vi "GUI_BELLA_CAP_PLC.vi"() -> ()   [LabVIEW 2013]
panel:
  out "OutPos_Sen":bool
  out "InPos_Sen":bool
  out "OutPos_Ctrl":bool
  out "InPos_Ctrl":bool
  in  "MoveOut":bool
  in  "stop":bool
  out "OutPos":bool
  out "InPos":bool
  in  "MoveIn":bool
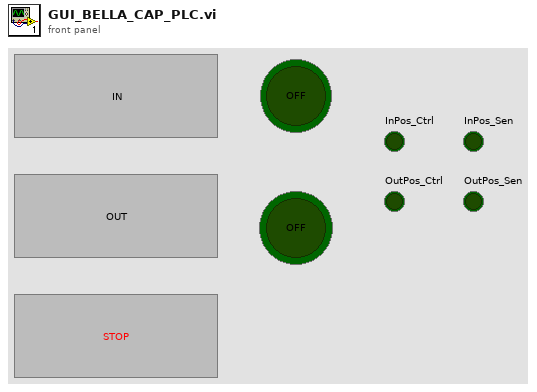
[diagram p1: front panel]
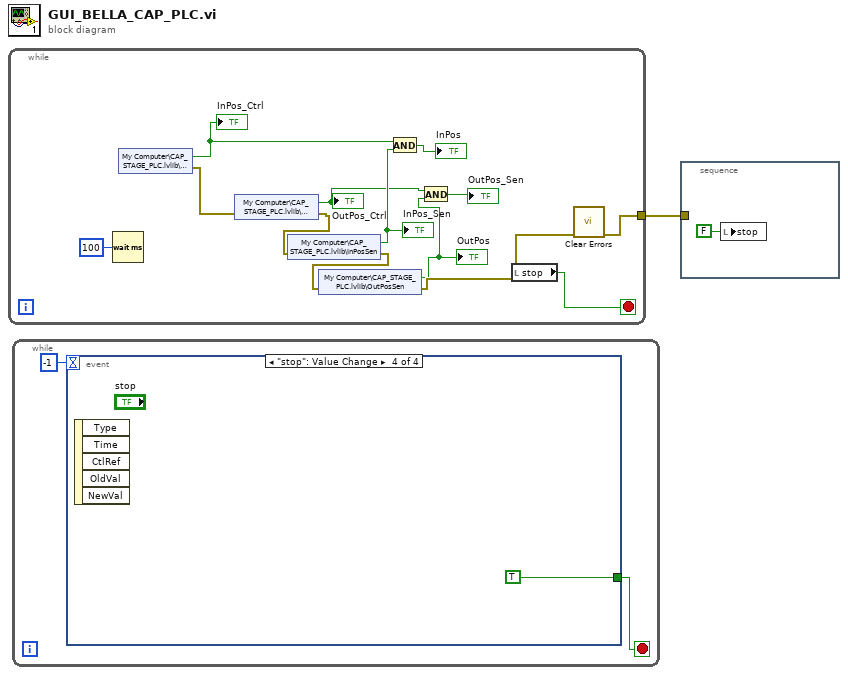
[diagram p0: block diagram]
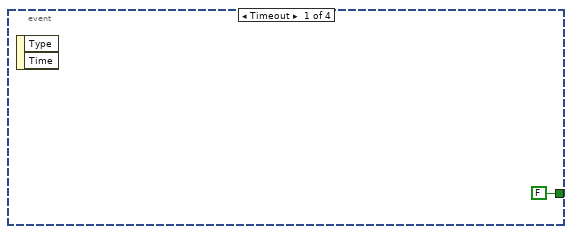
[diagram p2: hidden frame]
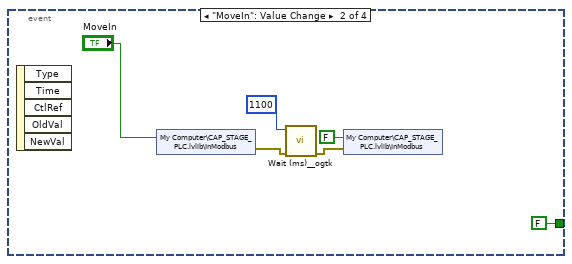
[diagram p3: hidden frame]
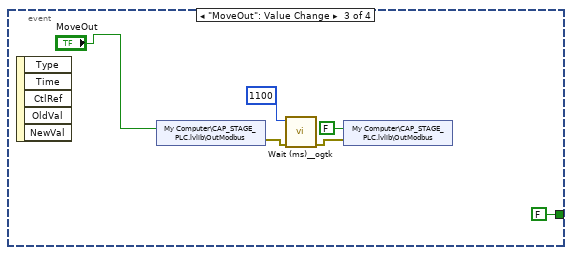
[diagram p4: hidden frame]
diagram:
  n1 = while {
    tunnel: [w11] -> w1
    stop <- w14 stop-if-true
    n2 = Wait (ms)(milliseconds to wait=u32 100) -> ()  [unwired: 1 out]
    n3 = shared-variable "My Computer\\CAP_STAGE_PLC.lvlib\\InPos"() -> (w6:bool, error out=w12:errorcluster)  [unwired: 1 in]
    "InPos_Ctrl" <- w6
    n4 = shared-variable "My Computer\\CAP_STAGE_PLC.lvlib\\OutPos"(error in=w12) -> (w3:bool, error out=w10:errorcluster)
    "OutPos_Ctrl" <- w3
    n5 = shared-variable "My Computer\\CAP_STAGE_PLC.lvlib\\InPosSen"(error in=w10) -> (w7:bool, error out=w9:errorcluster)
    "InPos_Sen" <- w7
    n6 = shared-variable "My Computer\\CAP_STAGE_PLC.lvlib\\OutPosSen"(error in=w9) -> (w4:bool, error out=w8:errorcluster)
    "OutPos" <- w4
    n7 = And(x=w6, y=w7) -> (x .and. y?=→"InPos":bool)
    n8 = And(x=w3, y=w4) -> (x .and. y?=→"OutPos_Sen":bool)
    n9 = local read "stop"() -> (w14:bool)
    n10 = call <vilib>:"Clear Errors.vi"("error in (no error)"=w8) -> ("error out"=w11:errorcluster)  [unwired: 6 in]
  }
  n11 = while {
    stop <- w15 stop-if-true
    n12 = event shown="[3] \"stop\": Value Change" {
      selector: _ -> [_ _ _ _]
      dyn-events: _ -> [_ _ _ _]
      timeout: -1 -> [_ _ _ _]
      tunnel: [FALSE FALSE FALSE TRUE] -> w15
      event Timeout {
        n13 = event-data() -> ()  [unwired: 1 in, 2 out]
      }
      event "MoveIn": Value Change {
        n14 = event-data() -> ()  [unwired: 1 in, 5 out]
        n15 = shared-variable "My Computer\\CAP_STAGE_PLC.lvlib\\InModbus"("MoveIn") -> (error out=w21:errorcluster)  [unwired: 1 in]
        n16 = call <userlib>:"Wait (ms)__ogtk.vi"("error in (no error)"=w21, "milliseconds to wait"=u32 1100) -> ("error out"=w19:errorcluster)  [unwired: 8 in, 1 out]
        n17 = shared-variable "My Computer\\CAP_STAGE_PLC.lvlib\\InModbus"(FALSE ("InModbus"), error in=w19) -> ()  [unwired: 1 out]
      }
      event "MoveOut": Value Change {
        n18 = event-data() -> ()  [unwired: 1 in, 5 out]
        n19 = shared-variable "My Computer\\CAP_STAGE_PLC.lvlib\\OutModbus"("MoveOut") -> (error out=w28:errorcluster)  [unwired: 1 in]
        n20 = call <userlib>:"Wait (ms)__ogtk.vi"("error in (no error)"=w28, "milliseconds to wait"=u32 1100) -> ("error out"=w26:errorcluster)  [unwired: 8 in, 1 out]
        n21 = shared-variable "My Computer\\CAP_STAGE_PLC.lvlib\\OutModbus"(FALSE ("InModbus"), error in=w26) -> ()  [unwired: 1 out]
      }
      event "stop": Value Change {
        n22 = event-data() -> ()  [unwired: 1 in, 5 out]
      }
    }
  }
  n23 = stacked-sequence {
    tunnel: w1 -> [_]
    frame #0 {
      n24 = local write "stop"(FALSE ("stop")) -> ()
    }
  }
